vi "date_path_h5.vi"(7 "Bases":path[](array[path]), 9 "SEQ File":path caption="SEQ File (*.osq)", 10 "time stamp":timestamp) -> (1 "RID":string, 2 "H5":path[](array[path]))   [LabVIEW 2015, in "oskar_tools.lvlib"]
uses:
  <vilib>/UPVI/lvhdf5/attribute.llb/Simple H5Awrite (Variant).vi
  <vilib>/UPVI/lvhdf5/attribute.llb/LVH5A Operation.ctl
  <vilib>/UPVI/lvhdf5/attribute.llb/Simple H5Awrite.xnode
  <vilib>/UPVI/lvhdf5/library.llb/HDF5 Ref.ctl
  oskar_tools.lvlib
panel:
  out "error out":errorcluster
  in  "error in":errorcluster
  in  "Save":bool=TRUE
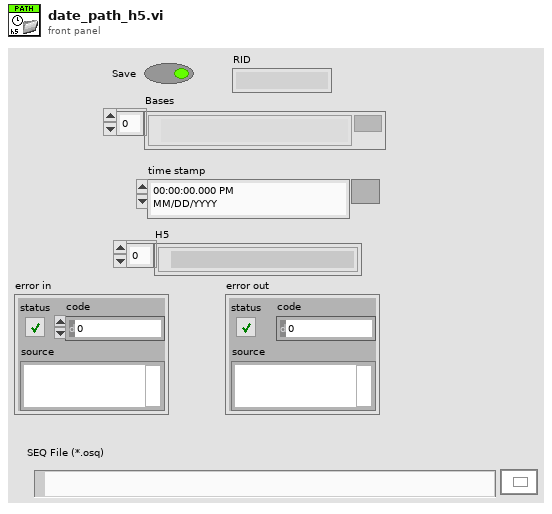
[diagram p1: front panel]
types:
  T1 = typedef "Semaphore RefNum" = refnum<k1>
  T2 = typedef "HDF5 Ref.ctl" = refnum<k1>
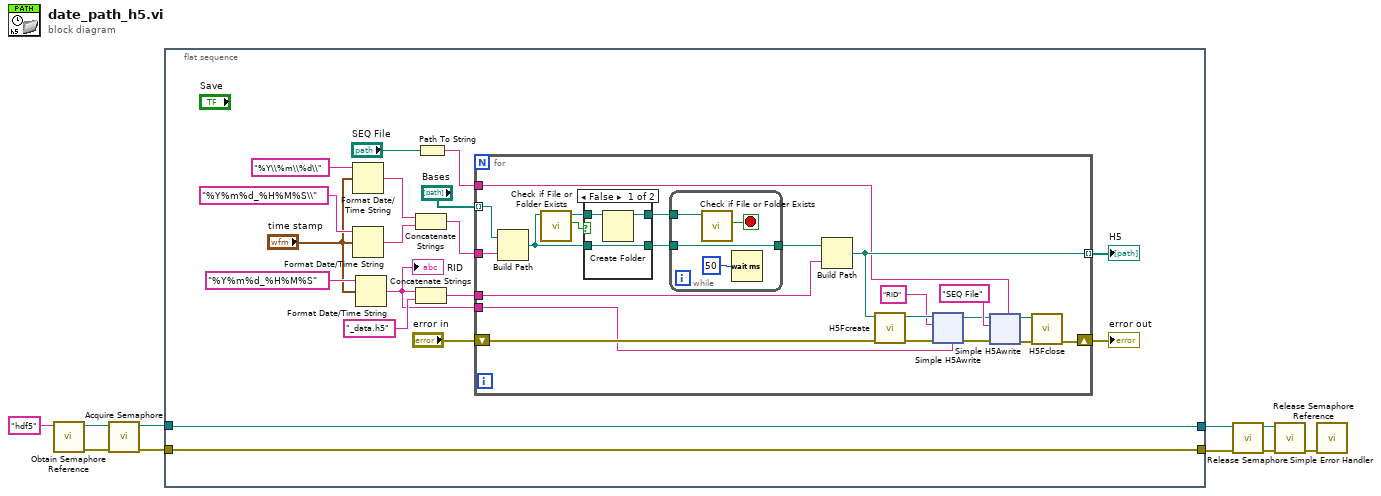
[diagram p0: block diagram]
diagram:
  n1 = call <vilib>:"Obtain Semaphore Reference.vi"("name (unnamed)"="hdf5") -> ("error out"=w9:errorcluster, "semaphore"=w10:T1)  [unwired: 4 in, 1 out]
  n2 = call <vilib>:"Acquire Semaphore.vi"("error in (no error)"=w9, "semaphore"=w10) -> ("error out"=w7:errorcluster, "semaphore out"=w6:T1)  [unwired: 3 in, 1 out]
  n3 = flat-sequence {
    tunnel: w7 -> [w12]
    tunnel: w6 -> [w11]
    tunnel: [w12] -> w2
    tunnel: [w11] -> w1
    frame #0 {
      n4 = Format Date/Time String(time format string (%c)="%Y\\%m\\%d\\", seconds (now)="time stamp") -> (date/time string=w27:string)  [unwired: 1 in]
      n5 = Format Date/Time String(time format string (%c)="%Y%m%d_%H%M%S\\", seconds (now)="time stamp") -> (date/time string=w24:string)  [unwired: 1 in]
      n6 = Format Date/Time String(time format string (%c)="%Y%m%d_%H%M%S", seconds (now)="time stamp") -> (date/time string=w15:string)  [unwired: 1 in]
      "RID" <- w15
      n7 = Concatenate Strings(w27, w24) -> (w26:string)
      n8 = Concatenate Strings(w15, "_data.h5" ("string")) -> (w18:string)
      n9 = Path To String(path="SEQ File") -> (string=w13:string)
      n10 = for {
        tunnel: w26 -> [w50]
        tunnel: "Bases" -> [w45] mode=indexing
        tunnel: [w40] -> w20 mode=indexing
        tunnel: w18 -> [w42]
        shift-right: [w30] -> w16
        shift-left: "error in" -> [w41]
        tunnel: w15 -> [w36]
        tunnel: w13 -> [w32]
        n11 = Build Path(base path=w45, name or relative path=w50) -> (appended path=w44:path)
        n12 = call <vilib>:"Check if File or Folder Exists.vi"("path"=w44) -> ("file or folder exists?"=w49:bool, "dup path"=w48:path)  [unwired: 8 in, 1 out]
        n13 = case shown="False" w49 {
          tunnel: w48 -> [w87 w88]
          tunnel: [w86 w89] -> w46
          tunnel: w44 -> [w86 w89]
          tunnel: [w85 w88] -> w47
          frame False {
            n14 = Create Folder(path (use dialog)=w87) -> (created path=w85:path)  [unwired: 2 in, 2 out]
          }
          frame True {
          }
        }
        n15 = while {
          tunnel: w47 -> [w83]
          tunnel: [w81] -> w43
          tunnel: w46 -> [w81]
          stop <- w84 stop-if-true
          n16 = call <vilib>:"Check if File or Folder Exists.vi"("path"=w83) -> ("file or folder exists?"=w84:bool)  [unwired: 8 in, 2 out]
          n17 = Wait (ms)(milliseconds to wait=u32 50) -> ()  [unwired: 1 out]
        }
        n18 = Build Path(base path=w43, name or relative path=w42) -> (appended path=w40:path)
        n19 = call <vilib>:"H5Fcreate.vi"("error in (no error)"=w41, "path"=w40) -> ("error out"=w39:errorcluster, "HDF5 Ref"=w38:T2)  [unwired: 6 in]
        n20 = xnode "Simple H5Awrite"("HDF5 Ref"=w38, "Name"="RID" ("attrib name"), "error in (no error)"=w39, "Value"=w36) -> ("HDF5 Ref out"=w33:T2, "error out"=w35:errorcluster)  [unwired: 1 in]
        n21 = xnode "Simple H5Awrite"("HDF5 Ref"=w33, "Name"="SEQ File" ("attrib name"), "error in (no error)"=w35, "Value"=w32) -> ("HDF5 Ref out"=w29:T2, "error out"=w31:errorcluster)  [unwired: 1 in]
        n22 = call <vilib>:"H5Fclose.vi"("error in (no error)"=w31, "HDF5 Ref"=w29) -> ("error out"=w30:errorcluster)  [unwired: 7 in]
      }
      "H5" <- w20
      "error out" <- w16
    }
  }
  n23 = call <vilib>:"Release Semaphore.vi"("error in (no error)"=w2, "semaphore"=w1) -> ("error out"=w5:errorcluster, "semaphore out"=w4:T1)  [unwired: 4 in]
  n24 = call <vilib>:"Release Semaphore Reference.vi"("error in (no error)"=w5, "semaphore"=w4) -> ("error out"=w3:errorcluster)  [unwired: 8 in, 1 out]
  n25 = call <vilib>:"Simple Error Handler.vi"("error in (no error)"=w3) -> ()  [unwired: 4 in, 5 out]
